vi "P4CMD Dialog_BuildPortString.vi"(9 "Port:":refnum<vi>, 11 "Server:":refnum<vi>) -> (2 "port string":string)   [LabVIEW 2020, in "NI_SCC_P4CMD.lvlib"]
uses:
  <vilib>/SourceControl/Providers/P4CMD/NI_SCC_P4CMD.lvlib
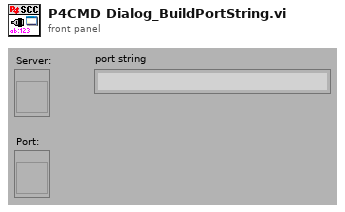
[diagram p1: front panel]
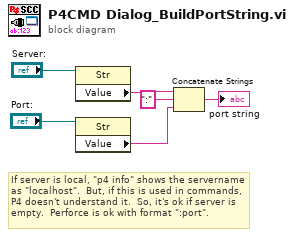
[diagram p0: block diagram]
diagram:
  # "If server is local, \"p4 info\" shows the servername as \"localhost\".  But, if this is used in commands, P4 doesn't understand it.  So, it's ok if server is empty.  Perforce is ok with format \":port\"."
  n1 = property class="Str"(reference="Server:") -> ("Value"=w6:string)  [unwired: 1 in, 2 out]
  n2 = property class="Str"(reference="Port:") -> ("Value"=w4:string)  [unwired: 1 in, 2 out]
  n3 = Concatenate Strings(w6, ":" ("string"), w4) -> (→"port string":string)
